vi "Year2017_Question2.vi"() -> ()   [LabVIEW 2015]
panel:
  in  "stop":bool
  out "Counter":dbl
  in  "Push Button":bool
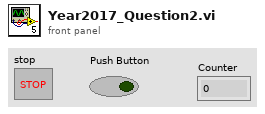
[diagram p1: front panel]
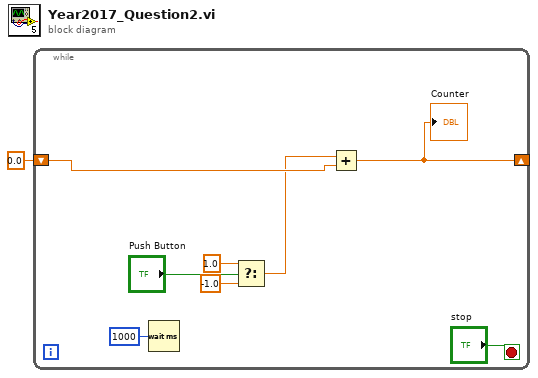
[diagram p0: block diagram]
diagram:
  n1 = while {
    shift-right: [w7] -> _
    shift-left: 0.0 -> [w9]
    stop <- "stop" stop-if-true
    n2 = Wait (ms)(milliseconds to wait=u32 1000) -> ()  [unwired: 1 out]
    n3 = Select(t=1.0, s="Push Button", f=-1.0) -> (s? t:f=w3:dbl)
    n4 = Add(x=w3, y=w9) -> (x+y=w7:dbl)
    "Counter" <- w7
  }
